vi "GetRectEnclosingPoints.vi"(8 "No Error":errorcluster, 9 "Clip":T1, 10 "Use Clip Rectangle (F)":bool, 11 "Points":T2[](array[typedef])) -> (0 "Error Out":errorcluster, 2 "Enclosing Rectangle":T1, 3 "Any Point Enclosed?":bool)   [LabVIEW 2024, in "SDL3.lvlib" / "Rect.lvlib"]
doc: "<B>Summary</B>\nCalculate a minimal rectangle enclosing a set of points.\n\n<B>Remarks</B>\nIf <B>Use Clip Rectangle</B> is true then only points inside of the clipping rectangle are considered."
uses:
  Rect.lvlib
  Rect--cluster.ctl
  Lib/SDL3.dll
  Point--cluster.ctl
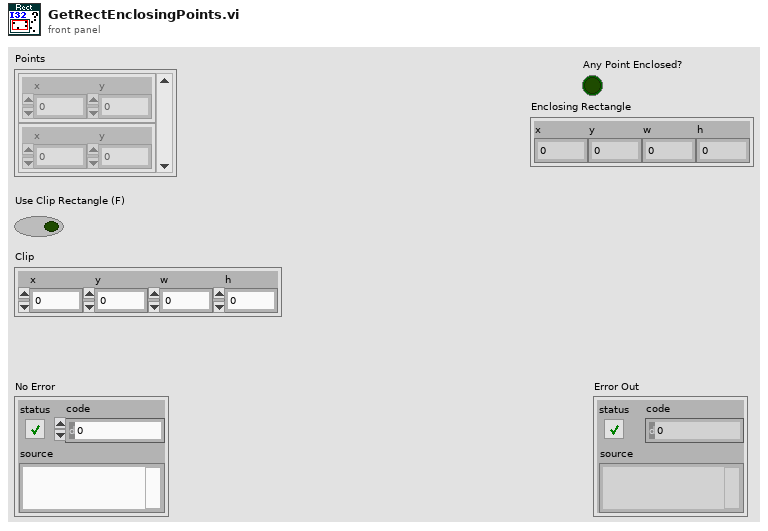
[diagram p1: front panel]
types:
  T1 = typedef "SDL3.lvlib/Rect.lvlib/Rect--cluster.ctl" = cluster{"x":i32, "y":i32, "w":i32, "h":i32}
  T2 = typedef "SDL3.lvlib/Rect.lvlib/Point--cluster.ctl" = cluster{"x":i32, "y":i32}
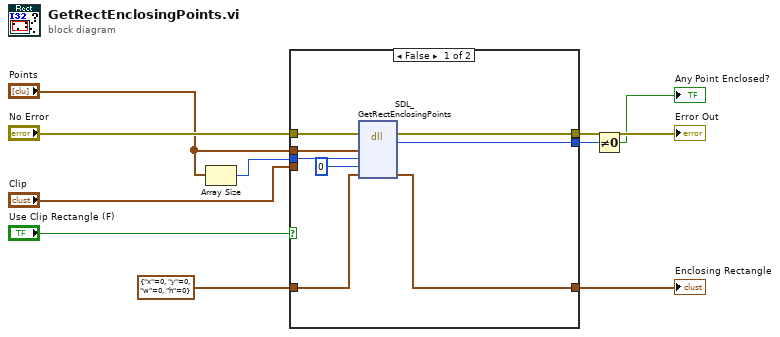
[diagram p0: block diagram]
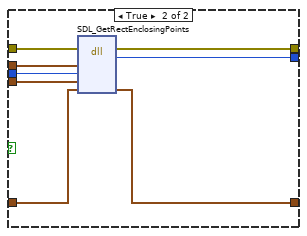
[diagram p2: hidden frame]
diagram:
  n1 = Array Size(array="Points") -> (size(s)=w3:i32)
  n2 = case shown="False" "Use Clip Rectangle (F)" {
    tunnel: "No Error" -> [w18 w26]
    tunnel: [w17 w25] -> w9
    tunnel: [w16 w24] -> w8
    tunnel: T1 {"x"=0, "y"=0, "w"=0, "h"=0} ("Enclosing Rectangle") -> [w15 w23]
    tunnel: [w14 w22] -> w5
    tunnel: "Points" -> [w13 w21]
    tunnel: w3 -> [w12 w20]
    tunnel: "Clip" -> [_ w19]
    frame False {
      n3 = dll-call lib="C:/Users/Thomas/Documents/Projects/LV-SDL3/Sources/SDL3/Lib/SDL3.*" fn="SDL_GetRectEnclosingPoints"(error in=w18, "points"=w13, "count"=w12, "clip"=i64 0, "result"=w15) -> (error out=w17:errorcluster, "return type"=w16:i32, "result"=w14:T1)  [unwired: 5 in, 1 out]
    }
    frame True {
      n4 = dll-call lib="C:/Users/Thomas/Documents/Projects/LV-SDL3/Sources/SDL3/Lib/SDL3.*" fn="SDL_GetRectEnclosingPoints"(error in=w26, "points"=w21, "count"=w20, "clip"=w19, "result"=w23) -> (error out=w25:errorcluster, "return type"=w24:i32, "result"=w22:T1)  [unwired: 5 in, 1 out]
    }
  }
  "Error Out" <- w9
  "Enclosing Rectangle" <- w5
  n5 = Not Equal To 0?(x=w8) -> (x != 0?=→"Any Point Enclosed?":bool)
